vi "DetermineNumberofPlanes.vi"(8 "error in (no error)":errorcluster, 11 "Z coordinates (pixels)":dbl[](array[numeric])) -> (0 "error out":errorcluster, 3 "number of planes to scan":i32)   [LabVIEW 2010]
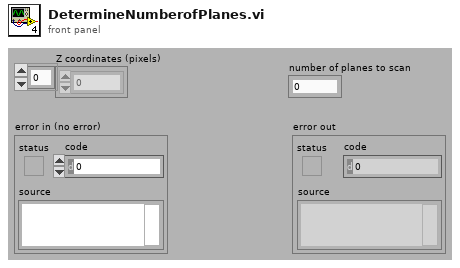
[diagram p1: front panel]
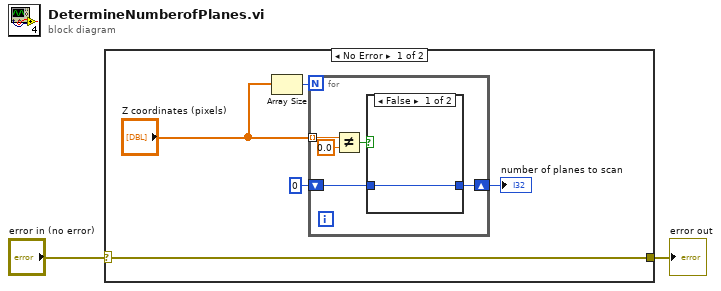
[diagram p0: block diagram]
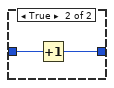
[diagram p2: hidden frame]
diagram:
  n1 = case shown="No Error" "error in (no error)" {
    selector: "error in (no error)" -> [w4 w16]
    tunnel: [w4 w16] -> w1
    frame No Error {
      n2 = Array Size(array="Z coordinates (pixels)") -> (size(s)=w7:i32)
      n3 = for {
        N: w7 -> [_]
        tunnel: "Z coordinates (pixels)" -> [w12] mode=indexing
        shift-right: [w8] -> w5
        shift-left: 0 ("dimension size") -> [w9]
        n4 = Not Equal?(x=w12, y=0.0) -> (x != y?=w10:bool)
        n5 = case shown="False" w10 {
          tunnel: w9 -> [w13 w15]
          tunnel: [w13 w14] -> w8
          frame False {
          }
          frame True {
            n6 = Increment(x=w15) -> (x+1=w14:i32)
          }
        }
      }
      "number of planes to scan" <- w5
    }
    frame Error {
    }
  }
  "error out" <- w1
